vi "Digitizer Fetch.vi"(4 "input impedance":u32(ring) items=["1 mega ohm"=0, "50 ohms"=2], 5 "Vertical Coupling":i32(ring)=1 items=["AC", "DC", "Ground"], 6 "Vertical Range (V)":dbl=2.0 format="%_3g", 7 "Pins":string[](array[string])=["Xout"], 8 "error in (no error)":errorcluster, 9 "Min Record Length":i32=1000 caption="Record Length", 10 "Min. Sample Rate":dbl=1000000.0 caption="Sample Rate" format="%#_6p", 11 "Semiconductor Module Context":T1) -> (0 "error out":errorcluster, 3 "Waveform Data Out":waveform(dbl)[](array[waveform]))   [LabVIEW 2014]
doc: "Example: Measurement Library\n\nRecommended Input Signal: 100 kHz, 2 Vpp, sine wave\n\nDevices Supported: Refer to NI Example Finders\n\nLabVIEW Description:\n\nThis example illustrates fetching scalar measurements from NI-SCOPE, such as period and rise time calculations. \n\nSome common horizontal and vertical parameters are configured for the oscilloscope. The property node is used to set the reference level units, and the low, middle and high reference levels. For more information about measurement library parameters, see the NI-SCOPE VI Reference Help file. \n\nAfter the Read VI is called to acquire a waveform, the Fetch Measurement Stats VI is used to perform the desired scalar measurement analysis on the waveform. NI-SCOPE keeps a history of each measurement's results, which allows it to retrieve the statistics computed over multiple acquisitions. These statistics include the mean, standard deviation, min, max and number of acquisitions used in the statistics. The statistics are updated once per acquisition when the measurement is fetched. The Clear Stats VI clears this history."
uses:
  <vilib>/NI_TestStand_SemiconductorModule/NI_TestStand_Semiconductor_Module.lvlibp/PinMap/General/SemiconductorModuleContext.ctl
  <vilib>/NI_TestStand_SemiconductorModule/NI_TestStand_Semiconductor_Module.lvlibp/PinMap/General/NIInstrumentTypeIDs.ctl
  <vilib>/NI_TestStand_SemiconductorModule/NI_TestStand_Semiconductor_Module.lvlibp/PinMap/Advanced/Custom Instruments/GetSessionData.vi
  <instrlib>/niScope/Configure/Trigger/niScope Configure Trigger Immediate.vi
  <instrlib>/niScope/Acquire/niScope Multi Read WDT.vi
  <vilib>/NI_TestStand_SemiconductorModule/NI_TestStand_Semiconductor_Module.lvlibp
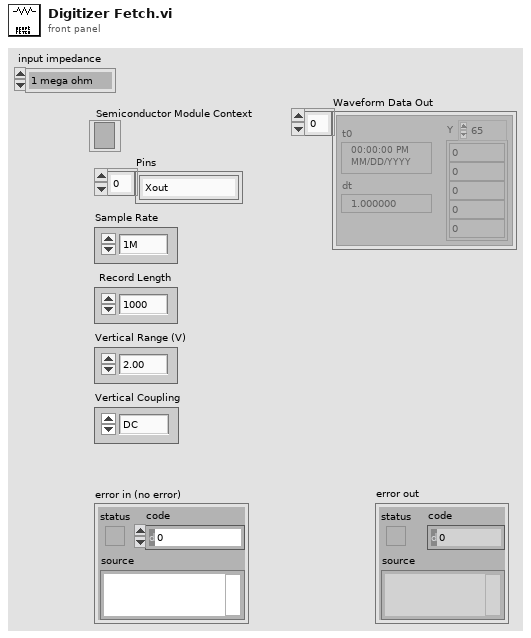
[diagram p1: front panel]
types:
  T1 = typedef "NI_TestStand_Semiconductor_Module.lvlibp/SemiconductorModuleContext.ctl" = refnum<k7>
  T2 = typedef "NI_TestStand_Semiconductor_Module.lvlibp/NIInstrumentTypeIDs.ctl" = string
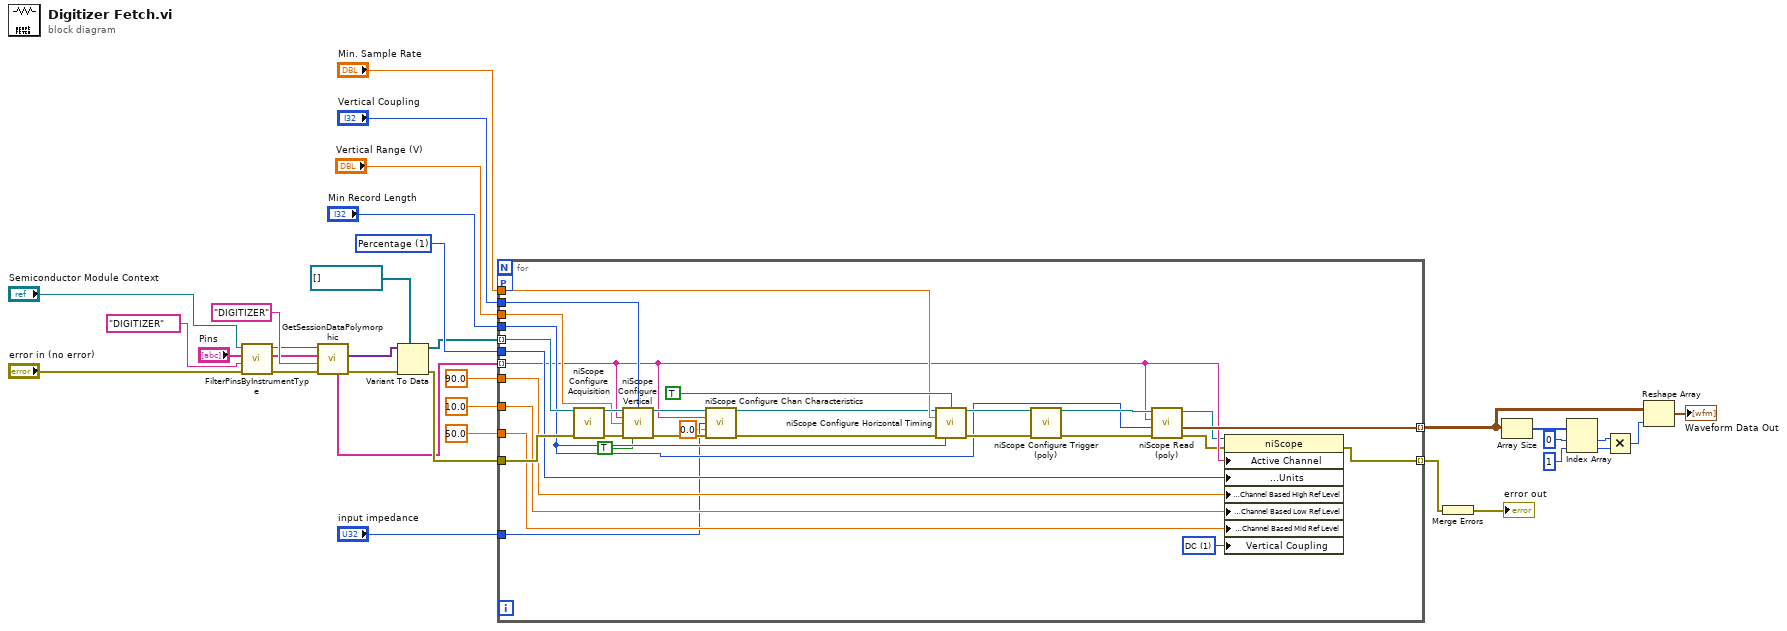
[diagram p0: block diagram]
diagram:
  w26 = u16 1 items=["Voltage", "Percentage"] ("Reference Level Units")
  n1 = call <vilib>:"FilterPinsByInstrumentType.vi"("error in (no error)"="error in (no error)", "Instrument Type Id"=T2 "DIGITIZER", "Pins"="Pins", "Semiconductor Module Context"="Semiconductor Module Context") -> ("error out"=w14:errorcluster, "Filtered Pins"=w13:string[], "Semiconductor Module Context Out"=w17:T1)  [unwired: 5 in]
  n2 = call-poly <vilib>:"GetSessionDataPolymorphic.vi"("error in (no error)"=w14, "Instrument Type Id"="DIGITIZER", "Pins"=w13, "Semiconductor Module Context"=w17) -> ("error out"=w32:errorcluster, "Session Data"=w31:variant[], "Channel Lists"=w5:string[])  [unwired: 2 in, 3 out]
  n3 = Variant To Data(error in=w32, type=refnum<k15>[] [], Variant=w31) -> (data=w22:refnum<k15>[], error out=w33:errorcluster)
  n4 = for {
    tunnel: "Min Record Length" -> [w48]
    tunnel: "Vertical Range (V)" -> [w57]
    tunnel: w5 -> [w40] mode=indexing
    tunnel: w26 -> [w56]
    tunnel: 90.0 ("High Ref.") -> [w55]
    tunnel: 10.0 ("Low Ref.") -> [w54]
    tunnel: 50.0 ("Mid Ref.") -> [w53]
    tunnel: w22 -> [w52] mode=indexing
    tunnel: "Min. Sample Rate" -> [w51]
    tunnel: "Vertical Coupling" -> [w45]
    tunnel: [w47] -> w12 mode=indexing
    tunnel: "input impedance" -> [w41]
    workers-P: _ -> [_]
    tunnel: w33 -> [w59]
    tunnel: [w34] -> w2 mode=indexing
    w44 = 1 items=["AC", "DC", "Ground"] ("Vertical:Vertical Coupling")
    n5 = call <instrlib>:"niScope Configure Acquisition.vi"("instrument handle"=w52, "error in"=w59) -> ("instrument handle out"=w62:refnum<k15>, "error out"=w63:errorcluster)  [unwired: 12 in]
    n6 = call <instrlib>:"niScope Configure Vertical.vi"("instrument handle"=w62, "vertical coupling"=w45, "channels"=w40, "vertical range"=w57, "error in"=w63, "channel enabled"=TRUE) -> ("instrument handle out"=w43:refnum<k15>, "error out"=w42:errorcluster)  [unwired: 8 in]
    n7 = call <instrlib>:"niScope Configure Chan Characteristics.vi"("instrument handle"=w43, "channels"=w40, "input impedance"=w41, "maximum input frequency"=0.0, "error in"=w42) -> ("instrument handle out"=w39:refnum<k15>, "error out"=w38:errorcluster)  [unwired: 9 in]
    n8 = call <instrlib>:"niScope Configure Horizontal Timing.vi"("instrument handle"=w39, "enforce realtime"=TRUE, "min sample rate"=w51, "error in"=w38, "min record length"=w48) -> ("instrument handle out"=w61:refnum<k15>, "error out"=w60:errorcluster)  [unwired: 9 in]
    n9 = call-poly <instrlib>:"niScope Configure Trigger (poly).vi"("instrument handle"=w61, "error in"=w60) -> ("instrument handle out"=w50:refnum<k15>, "error out"=w49:errorcluster)  [unwired: 12 in]
    n10 = call-poly <instrlib>:"niScope Read (poly).vi"("error in"=w49, "numSamples"=w48, "channels"=w40, "instrument handle"=w50) -> ("error out"=w36:errorcluster, "wfm"=w47:waveform(dbl)[], "instrument handle out"=w37:refnum<k15>)  [unwired: 4 in, 1 out]
    n11 = property class="niScope"(reference=w37, error in=w36, "Active Channel"=w40, "Waveform Measurement:Reference Levels:Units"=w56, "Waveform Measurement:Reference Levels:Channel Based High Ref Level"=w55, "Waveform Measurement:Reference Levels:Channel Based Low Ref Level"=w54, "Waveform Measurement:Reference Levels:Channel Based Mid Ref Level"=w53, "Vertical Coupling"=w44) -> (error out=w34:errorcluster)  [unwired: 1 out]
  }
  n12 = Merge Errors(w2) -> (→"error out":errorcluster)
  n13 = Array Size(array=w12) -> (size(s)=w11:i32[])
  n14 = Index Array(array=w11, index #1=0 ("index"), index #2=1 ("index")) -> (element #1=w8:i32, element #2=w7:i32)
  n15 = Multiply(x=w8, y=w7) -> (x*y=w6:i32)
  n16 = Reshape Array(w12, w6) -> (→"Waveform Data Out":waveform(dbl)[])
